vi "Handle Server Request.vi"(7 "parameters":string[][](array[string]), 8 "error in (no error)":errorcluster, 10 "id in":i32, 11 "request":string) -> (0 "error out":errorcluster, 3 "response":string)   [LabVIEW 2025, in "MCP Server.lvlib"]
doc: "Use this VI to handle an MCP RPC message. This VI accepts a json with request data and replies with a json object with response data. It implements the full MCP server. Use the MCP server api in your code to register tools and prompts and make them available in the server."
uses:
  MCP Server.lvlib
  <vilib>/JDP Science/JSONtext/LVClass Serializer/JSONtext LVClass Serializer.lvclass
  <vilib>/JDP Science/JSONtext/JSONtext.lvlib
  17ff933e-622e-44bb-904e-4e6adce09461.vi
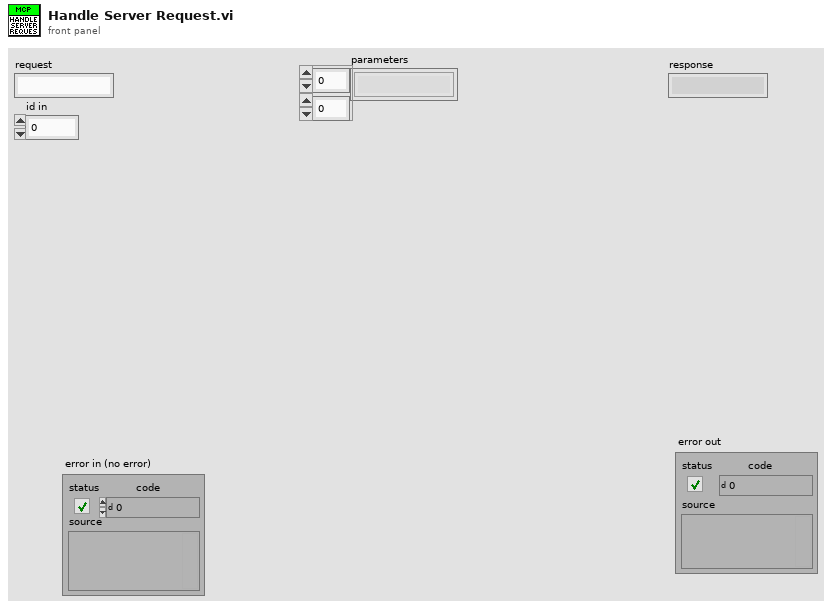
[diagram p1: front panel]
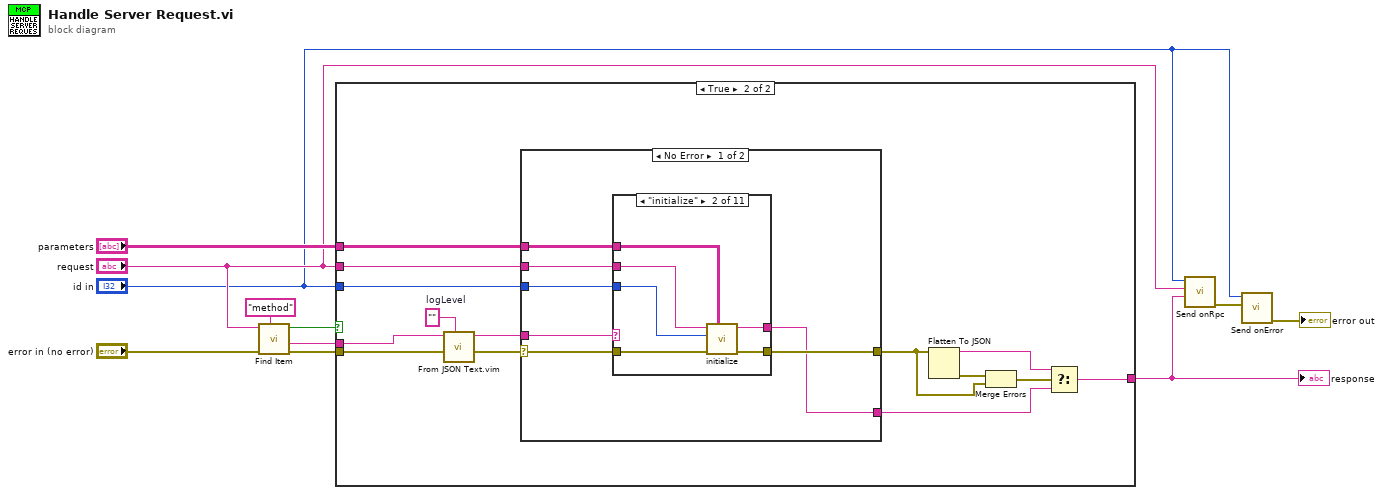
[diagram p0: block diagram]
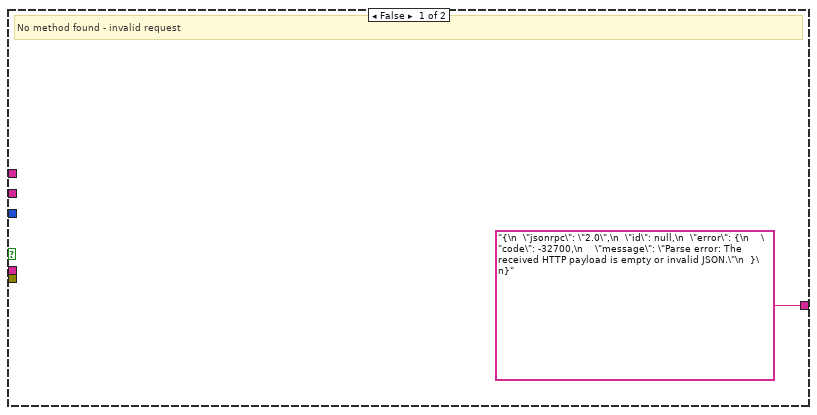
[diagram p2: hidden frame]
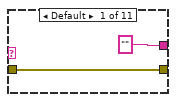
[diagram p3: hidden frame]
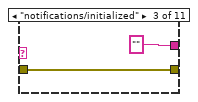
[diagram p4: hidden frame]
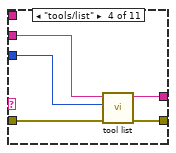
[diagram p5: hidden frame]
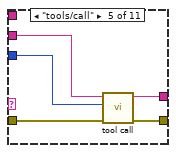
[diagram p6: hidden frame]
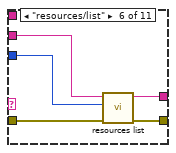
[diagram p7: hidden frame]
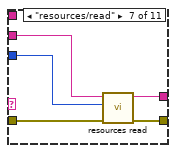
[diagram p8: hidden frame]
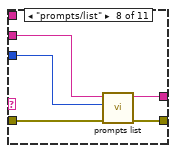
[diagram p9: hidden frame]
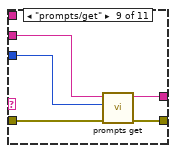
[diagram p10: hidden frame]
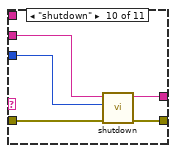
[diagram p11: hidden frame]
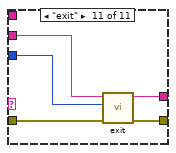
[diagram p12: hidden frame]
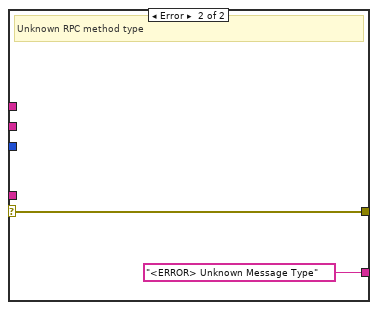
[diagram p13: hidden frame]
diagram:
  n1 = call <vilib>:"Find Item.vi"("$Path or Item Name"="method", "error in (no error)"="error in (no error)", "JSON"="request") -> ("error out"=w7:errorcluster, "<JSON>"=w8:string, "Found"=w1:bool)  [unwired: 5 in, 1 out]
  n2 = case shown="True" w1 {
    tunnel: "parameters" -> [_ w26]
    tunnel: w8 -> [_ w23]
    tunnel: w7 -> [_ w21]
    tunnel: "request" -> [_ w20]
    tunnel: "id in" -> [_ w18]
    tunnel: ["{\n  \"jsonrpc\": \"2.0\",\n  \"id\": null,\n  \"error\": {\n    \"code\": -32700,\n    \"message\": \"Parse error: The received HTTP payload is empty or invalid JSON.\"\n  }\n}" ("format string") w17] -> w2
    frame False {
      # "No method found - invalid request"
    }
    frame True {
      w22 = ""  # logLevel
      n3 = call "From JSON Text.vim"("Data Type and Default Value"=w22, "error in (no error)"=w21, "JSON"=w23) -> ("error out"=w24:errorcluster, "Data out"=w25:string)  [unwired: 7 in]
      n4 = case shown="No Error" w24 {
        selector: w24 -> [w32 w85]
        tunnel: w20 -> [w33 _]
        tunnel: [w31 w85] -> w15
        tunnel: [w30 "<ERROR> Unknown Message Type" ("response")] -> w19
        tunnel: w18 -> [w29 _]
        tunnel: w25 -> [w28 _]
        tunnel: w26 -> [w27 _]
        frame No Error {
          n5 = case shown="\"initialize\"" w28 {
            tunnel: w33 -> [_ w41 _ w48 w53 w58 w63 w68 w72 w78 w83]
            tunnel: ["" ("response") w40 "" ("response") w45 w50 w56 w61 w67 w70 w75 w80] -> w30
            tunnel: w32 -> [w35 w39 w43 w47 w52 w57 w62 w65 w73 w77 w82]
            tunnel: [w35 w38 w43 w46 w51 w55 w60 w66 w71 w76 w81] -> w31
            tunnel: w29 -> [_ w37 _ w44 w49 w54 w59 w64 w69 w74 w79]
            tunnel: w27 -> [_ w36 _ _ _ _ _ _ _ _ _]
            frame Default {
            }
            frame "initialize" {
              n6 = call "initialize.vi"("parameters"=w36, "error in"=w39, "server id"=w37, "message json"=w41) -> ("error out"=w38:errorcluster, "response"=w40:string)  [unwired: 6 in]
            }
            frame "notifications/initialized" {
            }
            frame "tools/list" {
              n7 = call "tool list.vi"("error in"=w47, "server id in"=w44, "message json"=w48) -> ("error out"=w46:errorcluster, "response"=w45:string)  [unwired: 7 in]
            }
            frame "tools/call" {
              n8 = call "tool call.vi"("error in"=w52, "id in"=w49, "message json"=w53) -> ("error out"=w51:errorcluster, "response"=w50:string)  [unwired: 7 in]
            }
            frame "resources/list" {
              n9 = call "resources list.vi"("error in"=w57, "server id"=w54, "message json"=w58) -> ("error out"=w55:errorcluster, "response"=w56:string)  [unwired: 7 in]
            }
            frame "resources/read" {
              n10 = call "resources read.vi"("error in"=w62, "id"=w59, "message json"=w63) -> ("error out"=w60:errorcluster, "response"=w61:string)  [unwired: 7 in]
            }
            frame "prompts/list" {
              n11 = call "prompts list.vi"("error in"=w65, "id"=w64, "message json"=w68) -> ("error out"=w66:errorcluster, "response"=w67:string)  [unwired: 7 in]
            }
            frame "prompts/get" {
              n12 = call "prompts get.vi"("error in"=w73, "id"=w69, "message json"=w72) -> ("error out"=w71:errorcluster, "response"=w70:string)  [unwired: 7 in]
            }
            frame "shutdown" {
              n13 = call "shutdown.vi"("error in"=w77, "id"=w74, "message json"=w78) -> ("error out"=w76:errorcluster, "response"=w75:string)  [unwired: 7 in]
            }
            frame "exit" {
              n14 = call "exit.vi"("error in"=w82, "id"=w79, "message json"=w83) -> ("error out"=w81:errorcluster, "response"=w80:string)  [unwired: 7 in]
            }
          }
        }
        frame Error {
          # "Unknown RPC method type"
        }
      }
      n15 = Flatten To JSON(anything=w15) -> (JSON string=w16:string, 11:w13:errorcluster)  [unwired: 2 in]
      n16 = Merge Errors(w13, w15) -> (w14:errorcluster)
      n17 = Select(t=w16, s=w14, f=w19) -> (s? t:f=w17:string)
    }
  }
  "response" <- w2
  n18 = call "Send onRpc.vi"("response"=w2, "request"="request", "id"="id in") -> ("error out"=w6:errorcluster)  [unwired: 8 in]
  n19 = call "Send onError.vi"("error to report"=w6, "id"="id in") -> ("error out"=→"error out":errorcluster)  [unwired: 9 in]
